vi "Instrument virtual pentru calculul modulului si fazei compo-nentelor spectrale folosind blocuri specializate.vi"() -> ()   [LabVIEW 2011]
uses:
  <vilib>/Analysis/NI_AALBase.lvlib
  <vilib>/Analysis/NI_AALPro.lvlib
  <vilib>/Analysis/0measdsp.llb/Scaled Time Domain Window (DBL).vi
  <vilib>/ptbypt/NI_PtbyPt.lvlib
panel:
  in  "Enum":enum16{""}(ring)
  in  "Boolean":bool
  in  "phase":dbl
  in  "window":enum8{"0", "1", "2", "3", ""}(ring)
  in  "display unit":enum8{"0", "1", "2", "3", ""}(ring)
  in  "log/linear":enum8{"0", "1"}(ring)
  in  "frequency":dbl
  in  "amplitude":dbl
  in  "Samples":i8
  out "Triangle Waze":dbl[](graph)
  out "Phase":T1(graph)
  out "Amplitude Spectrum":cluster{dbl, "df":dbl, "Spectrum out":dbl[]}(graph)
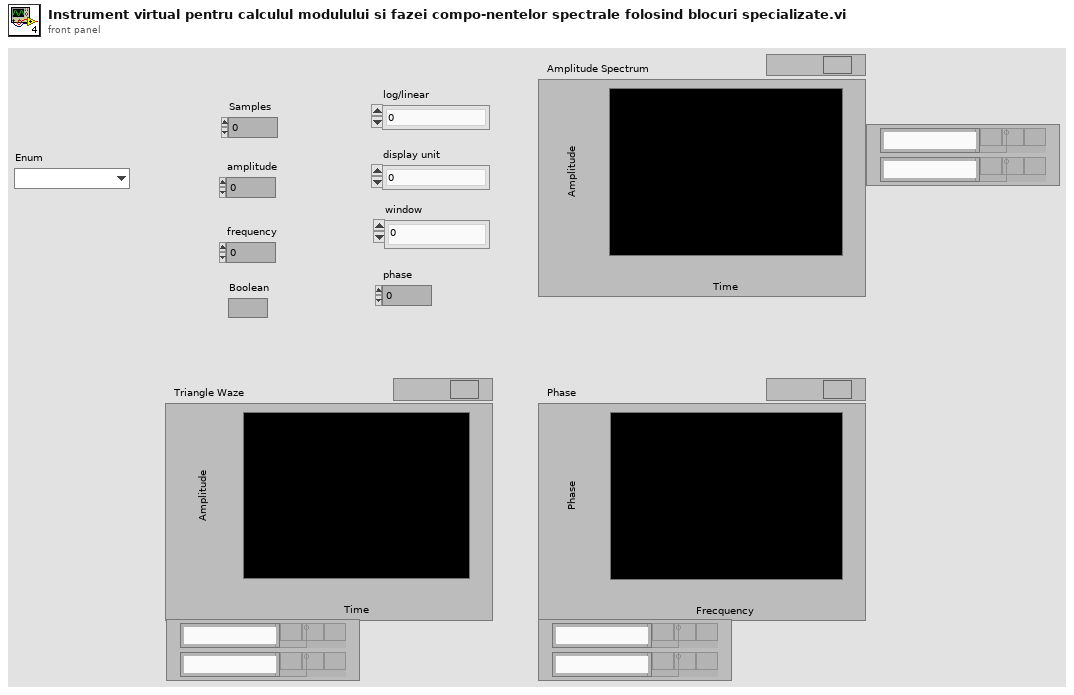
[diagram p1: front panel]
types:
  T1 = cluster{dbl, "df":dbl, "Amp Spectrum Phase (radians)":dbl[]}
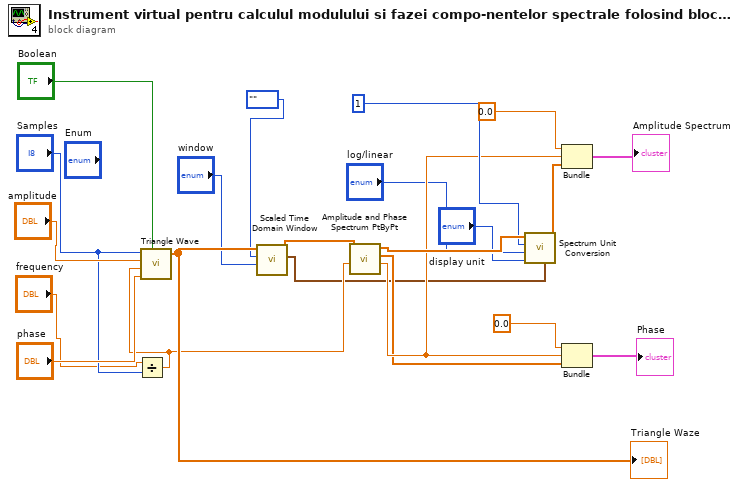
[diagram p0: block diagram]
diagram:
  n1 = Divide(x="frequency", y="Samples") -> (x/y=w16:dbl)
  n2 = call <vilib>:"Triangle Wave.vi"("samples"="Samples", "amplitude"="amplitude", "frequency"=w16, "phase in"="phase", "reset phase"="Boolean") -> ("triangle wave"=w17:dbl[])  [unwired: 2 out]
  "Triangle Waze" <- w17
  n3 = call-poly <vilib>:"Scaled Time Domain Window.vi"("window parameter"="window", "window"=enum16{""}."", "X"=w17) -> ("window properties"=w3:cluster{"eq noise BW":dbl, "coherent gain":dbl}, "Windowed X"=w6:dbl[])  [unwired: 6 in, 1 out]
  n4 = call <vilib>:"Amplitude and Phase Spectrum PtByPt.vi"("dt"=w16, "signal"=w6) -> ("df"=w10:dbl, "Amp Spectrum Phase (radians)"=w7:dbl[], "Amp Spectrum Mag (Vrms)"=w15:dbl[])  [unwired: 3 in, 1 out]
  n5 = call <vilib>:"Spectrum Unit Conversion.vi"("window constants"=w3, "display unit"="display unit", "log/linear"="log/linear", "spectrum type"=1 ("Spectrum type"), "Spectrum in"=w15) -> ("Spectrum out"=w14:dbl[])  [unwired: 5 in, 1 out]
  n6 = Bundle(0.0, "df"=w10, "Spectrum out"=w14) -> (→"Amplitude Spectrum":cluster{dbl, "df":dbl, "Spectrum out":dbl[]})  [unwired: 1 in]
  n7 = Bundle(0.0, "df"=w10, "Amp Spectrum Phase (radians)"=w7) -> (→"Phase":T1)  [unwired: 1 in]
